vi "onCheckConnection.vi"(8 "error in (no error)":errorcluster, 11 "LocalQueueConnection in":refnum<class "LocalQueueConnection.lvclass">) -> (0 "error out":errorcluster, 2 "connection OK":bool, 3 "LocalQueueConnection out":refnum<class "LocalQueueConnection.lvclass">)   [LabVIEW 2013, in "MQTT_Queue.lvlib" / "LocalQueueConnection.lvclass"]
uses:
  LocalQueueConnection.lvclass
  <vilib>/LabVIEW Open Source Project/MQTT Connection/MQTT_Connection/Connection/Connection.lvclass
  LocalQueueConnection.lvclass/LocalQueueConnection.ctl
  <vilib>/Utility/error.llb/Error Cluster From Error Code.vi
  <vilib>/ErrorRing/Error Ring.xnode
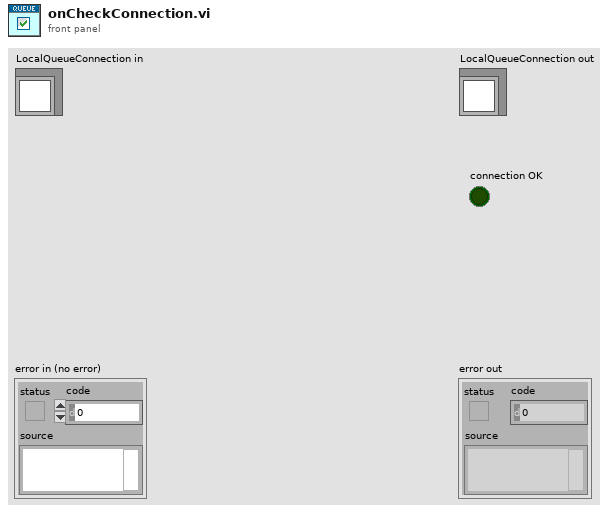
[diagram p1: front panel]
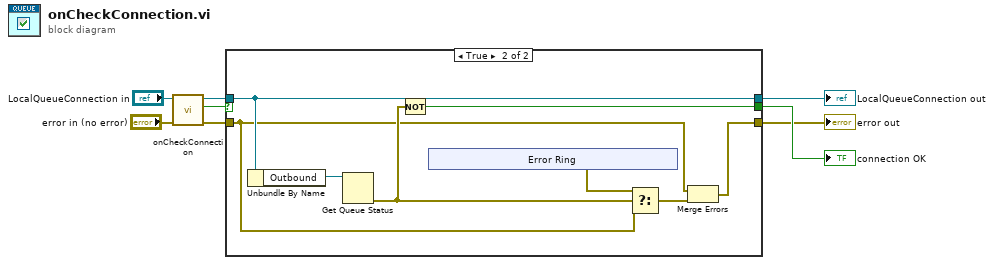
[diagram p0: block diagram]
diagram:
  n1 = call-parent "onCheckConnection.vi"("error in (no error)"="error in (no error)", "Connection in"="LocalQueueConnection in") -> ("error out"=w2:errorcluster, "connection OK"=w5:bool, "Connection out"=w6:refnum<class "LocalQueueConnection.lvclass">)  [unwired: 7 in]
  n2 = case shown="True" w5 {
    selector: w5 -> [w11 _]
    tunnel: w6 -> [w10 w18]
    tunnel: [w11 w17] -> w4
    tunnel: [w10 w18] -> w3
    tunnel: w2 -> [w9 w15]
    tunnel: [w9 w14] -> w1
    frame False {
    }
    frame True {
      n3 = Unbundle By Name(w18) -> ("Outbound"=w19:refnum<queue>)
      n4 = Get Queue Status(queue=w19) -> (error out=w16:errorcluster)  [unwired: 2 in, 7 out]
      n5 = Not(x=w16) -> (.not. x?=w17:bool)
      n6 = xnode "Error Ring"() -> ("error out"=w12:errorcluster)
      n7 = Select(t=w12, s=w16, f=w15) -> (s? t:f=w13:errorcluster)
      n8 = Merge Errors(w15, w13) -> (w14:errorcluster)
    }
  }
  "error out" <- w1
  "LocalQueueConnection out" <- w3
  "connection OK" <- w4
